vi "3d_Splint_Display_Standalone.vi"() -> ()   [LabVIEW 2016]
panel:
  out "status":bool
  out "ModelView Matrix":sgl[][](array[numeric])
  in  "stop":bool
  in  "Sensor Values":dbl[](array[slide]) scale=0.0..100.0
  out "error out":errorcluster
  in  "error in":errorcluster
  in  "Rendering Type":enum16{"3D Window", "3D Off"}(ring)=enum."3D Off"
  in  "Camera Controller":enum16{"None", "Spherical", "Flying"}(ring)=enum."Spherical"
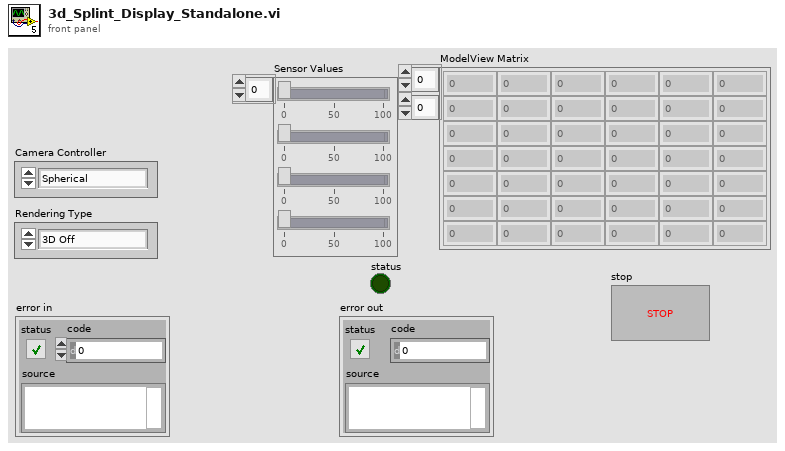
[diagram p1: front panel]
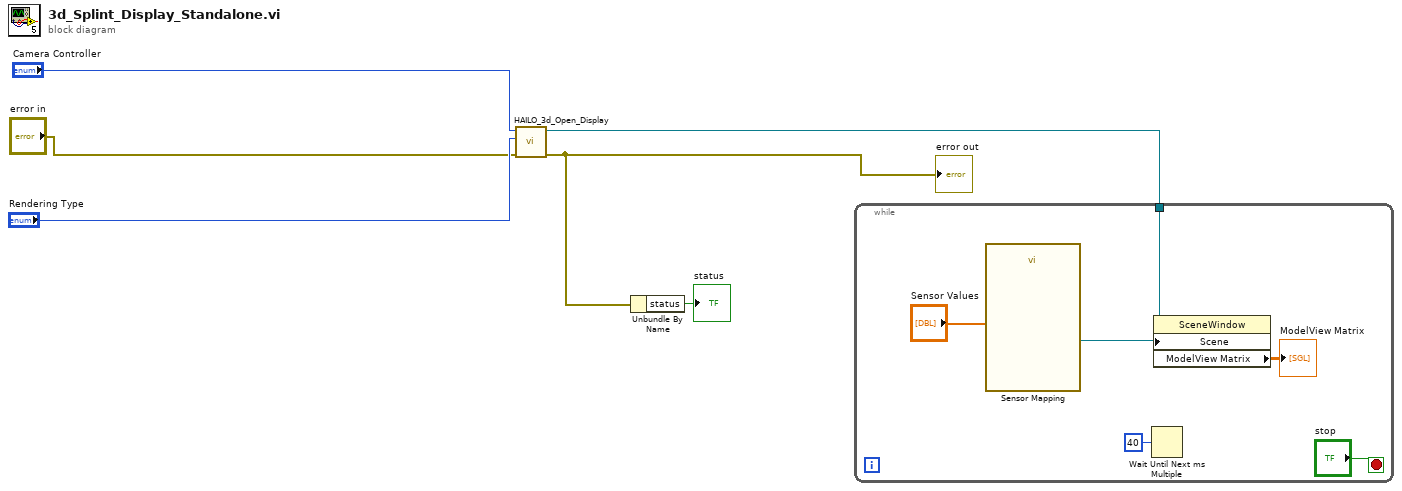
[diagram p0: block diagram]
diagram:
  n1 = call "HAILO_3d_Open_Display.vi"("error in (no error)"="error in", "Rendering Type"="Rendering Type", "Camera Controller"="Camera Controller") -> ("error out"=w2:errorcluster, "SceneWindow out"=w3:refnum<vi>)  [unwired: 7 in]
  "error out" <- w2
  n2 = Unbundle By Name(w2) -> ("status"=→"status":bool)
  n3 = while {
    tunnel: w3 -> [w10]
    stop <- "stop" stop-if-true
    n4 = call "Sensor Mapping"("Sensor Values"="Sensor Values") -> ("Scene Ref Out"=w12:refnum<vi>)  [unwired: 9 in, 1 out]
    n5 = Wait Until Next ms Multiple(millisecond multiple=u32 40) -> ()  [unwired: 1 out]
    n6 = property class="SceneWindow"(reference=w10, "Scene"=w12) -> ("ModelView Matrix"=→"ModelView Matrix":sgl[][])  [unwired: 1 in, 2 out]
  }
